vi "test_ini_remove_it.vi"(8 "error in":errorcluster {"code" format="%.0x"}, 11 "pulse_gen_and_detect_p2p out":refnum<class "pulse_gen_and_detect_p2p.lvclass">) -> (0 "error out":errorcluster, 3 "pulse_gen_and_detect_p2p out 2":refnum<class "pulse_gen_and_detect_p2p.lvclass">)   [LabVIEW 2021, in "pulse_gen_and_detect_p2p.lvclass"]
uses:
  pulse_gen_and_detect_p2p.lvclass
  <instrlib>/niRFSA/niRFSA.llb/niRFSA Acquisition Types.ctl
  pulse_gen_and_detect_p2p.lvclass/pulse_gen_and_detect_p2p.ctl
  <vilib>/FPGAPlugInAG/PXIe-5785 (KU060)/niLvFpga_Open_PXIe-5785 (KU060).vi
  <vilib>/rvi/interface/common/dynamic/niFpgaDynamicAddResources.vi
  <vilib>/FPGAPlugInAG/Dynamic/niLvFpga_P2PGetEndpoint_Dynamic.vi
  <vilib>/rvi/interface/nirviOpenFPGA/nirviOpenFPGA.xnode
  FPGA Bitfiles/5785_p2p_IQ_gen_1_6GHz_max_and_pulse_detector.lvbitx
  <vilib>/rvi/interface/nirviMethod/nirviMethod.xnode
  <vilib>/rvi/errors/niLvFpgaMergeErrorWithErrorCode.vi
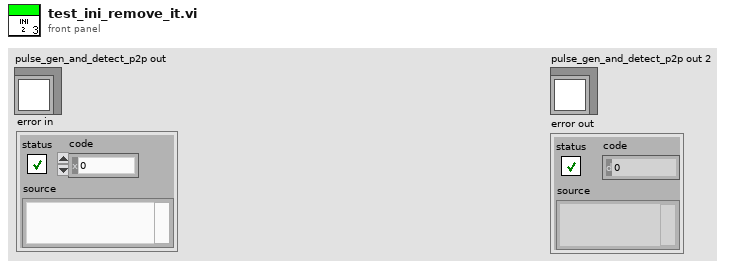
[diagram p1: front panel]
types:
  T1 = typedef "niRFSA Acquisition Types.ctl" = i32
  T2 = typedef "nirio_resource_hc.ctl" = tag
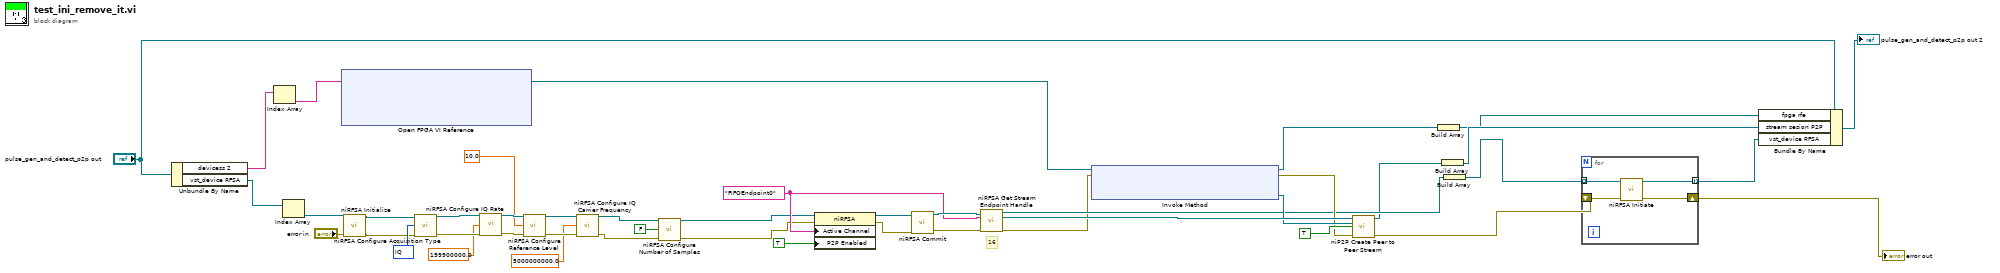
[diagram p0: block diagram]
diagram:
  w28 = "FIFOEndpoint0" ("Active Channel")
  w45 = T1 100 items=["IQ"=100, "Spectrum"=101] ("acquisition type")
  # "16"
  n1 = Unbundle By Name("pulse_gen_and_detect_p2p out") -> ("devicess 2"=w22:T2[], "vst_device RFSA"=w26:refnum<k15>[])
  n2 = Index Array(array=w22) -> (element=w21:T2)  [unwired: 1 in]
  n3 = Index Array(array=w26) -> (element=w25:refnum<k15>)  [unwired: 1 in]
  n4 = xnode "Open FPGA VI Reference"("resource name"=w21) -> ("FPGA VI Reference Out"=w20:refnum<k20>)  [unwired: 1 in, 1 out]
  n5 = call <instrlib>:"niRFSA Initialize.vi"("resource name"=w25, "error in"="error in") -> ("instrument handle out"=w44:refnum<k15>, "error out"=w43:errorcluster)  [unwired: 12 in]
  n6 = call <instrlib>:"niRFSA Configure Acquisition Type.vi"("instrument handle"=w44, "acquisition type"=w45, "error in"=w43) -> ("instrument handle out"=w34:refnum<k15>, "error out"=w31:errorcluster)  [unwired: 11 in]
  n7 = call <instrlib>:"niRFSA Configure IQ Rate.vi"("instrument handle"=w34, "IQ rate (S/s)"=199900000.0, "error in"=w31) -> ("instrument handle out"=w33:refnum<k15>, "error out"=w32:errorcluster)  [unwired: 11 in]
  n8 = call <instrlib>:"niRFSA Configure Reference Level.vi"("instrument handle"=w33, "reference level (dBm)"=10.0, "error in"=w32) -> ("instrument handle out"=w42:refnum<k15>, "error out"=w41:errorcluster)  [unwired: 11 in]
  n9 = call <instrlib>:"niRFSA Configure IQ Carrier Frequency.vi"("instrument handle"=w42, "carrier frequency"=5000000000.0, "error in"=w41) -> ("instrument handle out"=w4:refnum<k15>, "error out"=w3:errorcluster)  [unwired: 11 in]
  n10 = call <instrlib>:"niRFSA Configure Number of Samples.vi"("instrument handle"=w4, "number of samples is finite"=FALSE, "error in"=w3) -> ("instrument handle out"=w2:refnum<k15>, "error out"=w1:errorcluster)  [unwired: 11 in]
  n11 = property class="niRFSA"(reference=w2, error in=w1, "Active Channel"=w28, "P2P Enabled"=TRUE ("Peer-to-Peer:Enabled")) -> (reference out=w40:refnum<k15>, error out=w39:errorcluster)
  n12 = call <instrlib>:"niRFSA Commit.vi"("instrument handle"=w40, "error in"=w39) -> ("instrument handle out"=w38:refnum<k15>, "error out"=w37:errorcluster)  [unwired: 12 in]
  n13 = call <instrlib>:"niRFSA Get Stream Endpoint Handle.vi"("instrument handle"=w38, "stream endpoint"=w28, "error in"=w37) -> ("instrument handle out"=w16:refnum<k15>, "writer handle"=w36:refnum<k20>, "error out"=w11:errorcluster)  [unwired: 10 in]
  n14 = xnode "Invoke Method"("FPGA VI Reference In"=w20, "error in"=w11) -> ("FPGA VI Reference Out"=w12:refnum<k20>, "error out"=w18:errorcluster, "Reader"=w35:refnum<k20>)
  n15 = call <vilib>:"niP2P Create Peer to Peer Stream.vi"("writer"=w36, "reader"=w35, "enable stream (T)"=TRUE, "error in (no error)"=w18) -> ("stream session"=w14:refnum<k20>, "error out"=w9:errorcluster)  [unwired: 10 in]
  n16 = Build Array(w12) -> (w13:refnum<k20>[])
  n17 = Build Array(w14) -> (w15:refnum<k20>[])
  n18 = Build Array(w16) -> (w7:refnum<k15>[])
  n19 = for {
    tunnel: w7 -> [w49] mode=indexing
    shift-right: [w47] -> w8
    shift-left: w9 -> [w48]
    tunnel: [w46] -> w6 mode=indexing
    n20 = call <instrlib>:"niRFSA Initiate.vi"("instrument handle"=w49, "error in"=w48) -> ("instrument handle out"=w46:refnum<k15>, "error out"=w47:errorcluster)  [unwired: 12 in]
  }
  "error out" <- w8
  n21 = Bundle By Name(cluster="pulse_gen_and_detect_p2p out", "fpga rfe"=w13, "stream sesion P2P"=w15, "vst_device RFSA"=w6) -> (→"pulse_gen_and_detect_p2p out 2":refnum<class "pulse_gen_and_detect_p2p.lvclass">)
